vi "ReadMoxa8.vi"(0 "PORT 1":dbl, 1 "PORT 2":dbl, 3 "PORT 3":dbl, 4 "PORT 4":dbl, 5 "PORT 5":dbl, 6 "PORT 6":dbl, 10 "PORT 7":dbl, 12 "PORT 8":dbl, 16 "enable1":i32, 17 "enable2":i32, 18 "enable3":i32) -> (15 "params":dbl[](array[numeric]))   [LabVIEW 2017]
uses:
  BERTTA.dll
panel:
  # "int ports[12] = {1,2,4,3,6,5,8,0,0,0,0,0};"
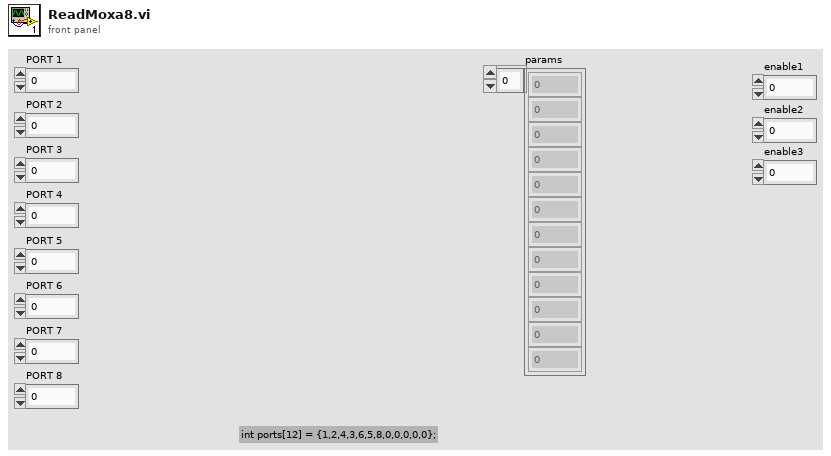
[diagram p1: front panel]
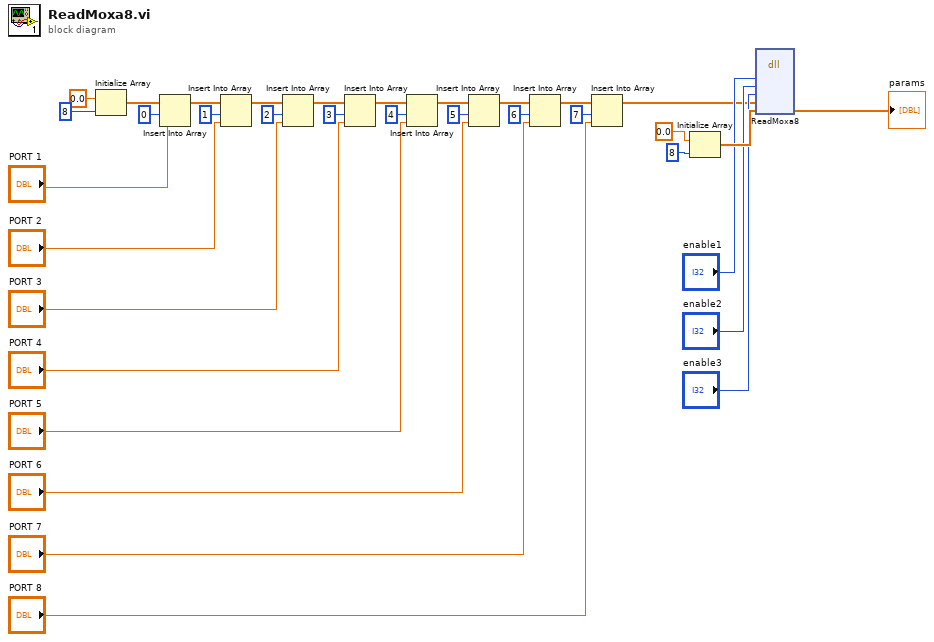
[diagram p0: block diagram]
diagram:
  n1 = Initialize Array(0.0 ("element"), 8 ("dimension size")) -> (w33:dbl[])
  n2 = Insert Into Array(array=w33, index=0, new element="PORT 1") -> (w31:dbl[])
  n3 = Insert Into Array(array=w31, index=1, new element="PORT 2") -> (w30:dbl[])
  n4 = Insert Into Array(array=w30, index=2, new element="PORT 3") -> (w29:dbl[])
  n5 = Insert Into Array(array=w29, index=3, new element="PORT 4") -> (w28:dbl[])
  n6 = Insert Into Array(array=w28, index=4, new element="PORT 5") -> (w27:dbl[])
  n7 = Insert Into Array(array=w27, index=5, new element="PORT 6") -> (w26:dbl[])
  n8 = Insert Into Array(array=w26, index=6, new element="PORT 7") -> (w25:dbl[])
  n9 = Insert Into Array(array=w25, index=7, new element="PORT 8") -> (w1:dbl[])
  n10 = Initialize Array(0.0 ("element"), 8 ("dimension size")) -> (w6:dbl[])
  n11 = dll-call lib="C:/Users/shresplab/OneDrive - Kemira Oyj/Documents/GitHub/Bertta/BERTTA/x64/Debug/BERTTA.dll" fn="ReadMoxa8"("enable1"="enable1", "enable2"="enable2", "enable3"="enable3", "ports"=w1, "params"=w6) -> ("params"=→"params":dbl[])  [unwired: 8 in, 2 out]
